vi "Copy_from_to_exp.vi"(8 "error in (no error)":errorcluster, 9 "Copy only data":bool, 10 "Experiment copy to":refnum<class "Experiment.lvclass">, 11 "Experiment copy from":refnum<class "Experiment.lvclass">) -> (0 "error out":errorcluster, 3 "Experiment copied":refnum<class "Experiment.lvclass">)   [LabVIEW 2020, in "Experiment.lvclass"]
uses:
  Experiment.lvclass
  Experiment.lvclass/Experiment.ctl
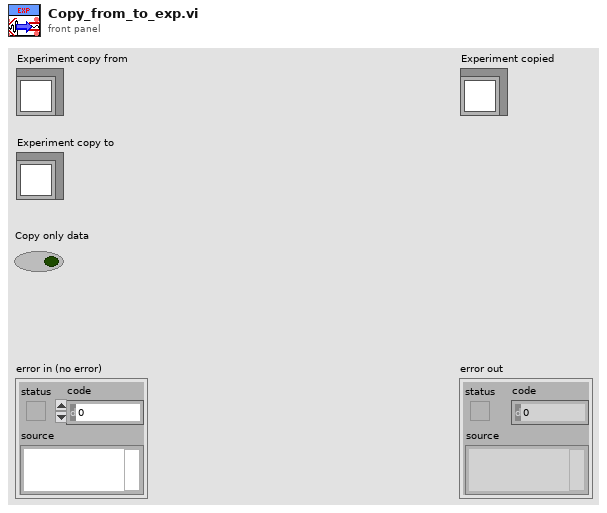
[diagram p1: front panel]
types:
  T1 = cluster{"From Time pix":i32, "To Time pix":i32, "From Wave pix":i32, "To Wave pix":i32}
  T2 = typedef "Oscilloscope.lvclass/Def_WCM_limits.ctl" = cluster{"WCM_min":dbl, "WCM_max":dbl, "WCM_set":dbl}
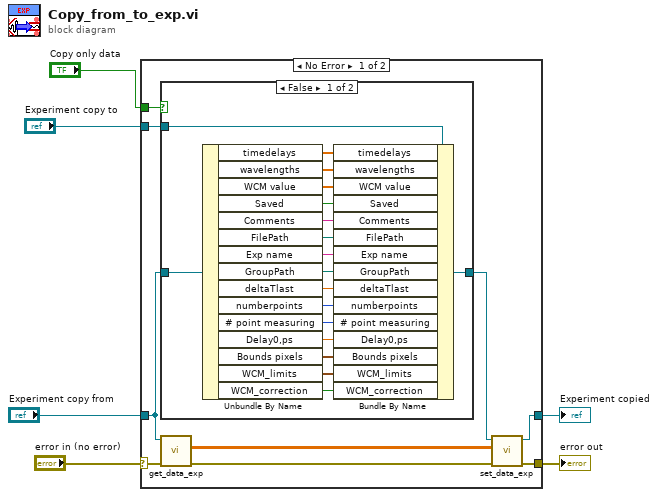
[diagram p0: block diagram]
diagram:
  n1 = case shown="No Error" "error in (no error)" {
    selector: "error in (no error)" -> [w14 w36]
    tunnel: [w8 w36] -> w5
    tunnel: [w9 w35] -> w3
    tunnel: "Experiment copy from" -> [w13 w35]
    tunnel: "Experiment copy to" -> [w15 _]
    tunnel: "Copy only data" -> [w7 _]
    frame No Error {
      n2 = case shown="False" w7 {
        tunnel: w15 -> [w33 w34]
        tunnel: w13 -> [w17 _]
        tunnel: [w16 w34] -> w11
        frame False {
          n3 = Unbundle By Name(w17) -> ("timedelays"=w18:dbl[], "wavelengths"=w19:dbl[], "WCM value"=w20:sgl[], "Saved"=w21:bool, "Comments"=w22:string, "FilePath"=w23:path, "Exp name"=w24:string, "GroupPath"=w25:path, "deltaTlast"=w26:dbl, "numberpoints"=w27:i32, "# point measuring"=w28:i32, "Delay0,ps"=w29:dbl, "Bounds pixels"=w30:T1, "WCM_limits"=w31:T2, "WCM_correction"=w32:bool)
          n4 = Bundle By Name(cluster=w33, "timedelays"=w18, "wavelengths"=w19, "WCM value"=w20, "Saved"=w21, "Comments"=w22, "FilePath"=w23, "Exp name"=w24, "GroupPath"=w25, "deltaTlast"=w26, "numberpoints"=w27, "# point measuring"=w28, "Delay0,ps"=w29, "Bounds pixels"=w30, "WCM_limits"=w31, "WCM_correction"=w32) -> (w16:refnum<class "Experiment.lvclass">)
        }
        frame True {
        }
      }
      n5 = call "get_data_exp.vi"("error in (no error)"=w14, "Experiment.lvclass in"=w13) -> ("error out"=w12:errorcluster, "Data"=w10:sgl[][])  [unwired: 7 in, 1 out]
      n6 = call "set_data_exp.vi"("error in (no error)"=w12, "Data"=w10, "Experiment.lvclass in"=w11) -> ("error out"=w8:errorcluster, "Experiment.lvclass out"=w9:refnum<class "Experiment.lvclass">)  [unwired: 7 in]
    }
    frame Error {
    }
  }
  "error out" <- w5
  "Experiment copied" <- w3
